vi "New Terminate Event.vi"(11 "error in (no error)":errorcluster) -> (4 "Exit Event Ref":T1, 6 "Exit Req Event Registration Ref":T2, 15 "error out":errorcluster)   [LabVIEW 2011, in "ART2 Test Panel.lvlib" / "TLB_Dependencies.lvlib"]
uses:
  TLB_Dependencies.lvlib
  Exit Req Event Registration Ref.ctl
  Exit Event Ref.ctl
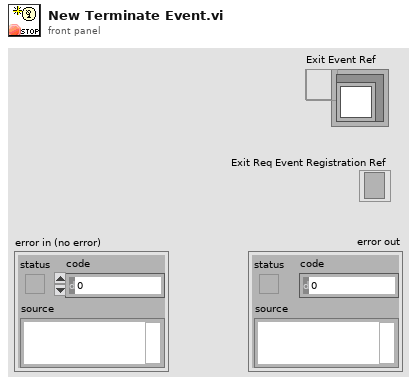
[diagram p1: front panel]
types:
  T1 = typedef "ART2 Test Panel.lvlib/TLB_Dependencies.lvlib/Exit Event Ref.ctl" = refnum<user-event>
  T2 = typedef "ART2 Test Panel.lvlib/TLB_Dependencies.lvlib/Exit Req Event Registration Ref.ctl" = refnum<event-registration>
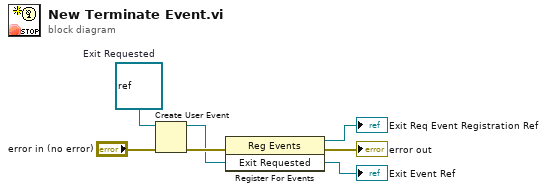
[diagram p0: block diagram]
diagram:
  w5 = refnum<class> refnum  # Exit Requested
  n1 = Create User Event(user event datatype=w5, error in="error in (no error)") -> (user event=w3:refnum<user-event>, error out=w6:errorcluster)
  "Exit Event Ref" <- w3
  n2 = register-events(error in=w6, w3) -> (reference out=→"Exit Req Event Registration Ref":refnum<event-registration>, error out=→"error out":errorcluster)  [unwired: 1 in]
